vi "Teleop.vi"(10 "Match Info":T1={"Autonomous Elapsed Seconds"=0.0, "TeleOp Elapsed Seconds"=0.0, "Disabled Elapsed Seconds"=0.0, "Visited Autonomous"=FALSE, "Visited TeleOp"=FALSE, "Visited Disabled"=FALSE, "Autonomous Settings"={"Autonomous Style"=enum."Independent", "VI Refnum"=refnum}}, 11 "Call Context":T2) -> ()   [LabVIEW 2016]
doc: "This VI is called for each TeleOp packet received from the DS where the robot is not disabled. It is often used to read from the joysticks and update I/O or to update setpoints for timed control loops. It should complete and return within 20 milliseconds or it may miss DS packets."
uses:
  <vilib>/Rock Robotics/WPI/DriverStation/WPI_DriverStationDerivedRobotMode.ctl
  <vilib>/Rock Robotics/WPI/DriverStation/WPI_DriverStationMatch Info.ctl
  <vilib>/Rock Robotics/WPI/Solenoid/WPI_SolenoidValue.ctl
  <vilib>/Rock Robotics/Network Tables/NT Read Boolean.vi
  <vilib>/Rock Robotics/Network Tables/NT Read Number.vi
  <vilib>/Rock Robotics/WPI/Utilities/WPI_GetSetVariantRefNum.vi
  <vilib>/Rock Robotics/WPI/Solenoid/WPI_SolenoidSetEnum.vi
panel:
  in  "Reset":bool
  out "Teleop Time Elipsed":dbl
  in  "Quand arreter compresseur":dbl
  out "Droit":dbl
  out "Gauche":dbl
  out "Corde start time":dbl
  out "Sample Slider 0":dbl(slide) scale=0.0..5.0
  out "Sample Boolean 1":bool
  out "Sample Boolean 0":bool
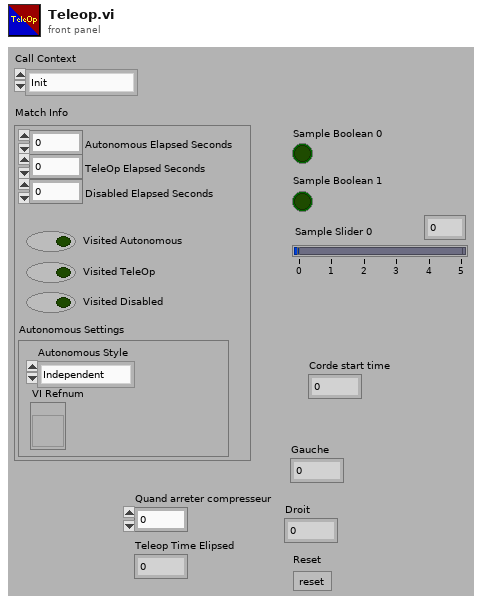
[diagram p1: front panel]
types:
  T1 = typedef "WPI_DriverStationMatch Info.ctl" = cluster{"Autonomous Elapsed Seconds":dbl, "TeleOp Elapsed Seconds":dbl, "Disabled Elapsed Seconds":dbl, "Visited Autonomous":bool, "Visited TeleOp":bool, "Visited Disabled":bool, "Autonomous Settings":cluster{"Autonomous Style":enum16{"Iterative", "Independent"}, "VI Refnum":refnum<vi>}}
  T2 = typedef "WPI_DriverStationDerivedRobotMode.ctl" = enum16{"Init", "Execute", "Stop"}
  T3 = typedef "WPI_SolenoidValue.ctl" = enum16{"Off", "On", "Forward", "Reverse"}
  T4 = typedef "WPI_JoystickDevRef.ctl" = cluster{"Device":T5}
  T5 = typedef "WPI_JoystickDeviceEnum.ctl" = enum16{"USB 0", "USB 1", "USB 2", "USB 3", "USB 4", "USB 5"}
  T6 = typedef "WPI_EncoderDevRef.ctl" = cluster{"DevStatus":errorcluster, "EncoderIndex":T7, "CounterIndex":T8, "DistancePerCount":dbl, "Decoding Type":T9}
  T7 = typedef "FPGA_EncoderIdx.ctl" = enum8{"Enc 0", "Enc 1", "Enc 2", "Enc 3", "Enc 4", "Enc 5", "Enc 6", "Enc 7", "Invalid"}
  T8 = typedef "FPGA_CounterCtrSystemIndex.ctl" = enum8{"Ctr 0", "Ctr 1", "Ctr 2", "Ctr 3", "Ctr 4", "Ctr 5", "Ctr 6", "Ctr 7", "Invalid"}
  T9 = typedef "WPI_EncoderType.ctl" = enum16{"1x", "2x", "4x"}
  T10 = cluster{"Buttons[0]":bool, "Buttons[1]":bool, "Buttons[2]":bool, "Buttons[3]":bool, "Buttons[4]":bool, "Buttons[5]":bool, "Buttons[6]":bool, "Buttons[7]":bool, "Buttons[8]":bool}
  T11 = cluster{"Axes[0]":dbl, "Axes[1]":dbl, "Axes[2]":dbl, "Axes[3]":dbl, "Axes[4]":dbl, "Axes[5]":dbl, "Axes[6]":dbl, "Axes[7]":dbl, "Axes[8]":dbl}
  T12 = typedef "WPI_MotorControlDeviceRef.ctl" = cluster{"DeviceStatus":errorcluster, "Type":T13, "PWM":cluster{"PWM Channel":T14, "DeadBand":T15}, "CAN":cluster{"Device Number":u8, "SetOutput VI Ref":variant, "GetOutput VI Ref":variant, "Enable VI Ref":variant, "Disable VI Ref":variant, "Data":variant}, "Invert":bool}
  T13 = typedef "WPI_MotorControlType.ctl" = enum16{"PWM", "CAN"}
  T14 = typedef "FPGA_DIOPWMChannel.ctl" = enum8{"PWM 0", "PWM 1", "PWM 2", "PWM 3", "PWM 4", "PWM 5", "PWM 6", "PWM 7", "PWM 8", "PWM 9", "PWM MXP 0", "PWM MXP 1", "PWM MXP 2", "PWM MXP 3", "PWM MXP 4", "PWM MXP 5", "PWM MXP 6", "PWM MXP 7", "PWM MXP 8", "PWM MXP 9", "Invalid"}
  T15 = typedef "WPI_PWMDeadband.ctl" = cluster{"Name":string, "maxPositivePwm":i32, "minPositivePwm":i32, "centerPwm":i32, "maxNegativePwm":i32, "minNegativePwm":i32, "angularRange":u16}
  T16 = typedef "WPI_SolenoidDevRef.ctl" = cluster{"DevStatus":errorcluster, "Pneumatics Control Module":u8, "Forward Solenoid Channel":T17, "Reverse Solenoid Channel":T17}
  T17 = typedef "WPI_SolenoidChannel.ctl" = enum8{"Solenoid 0", "Solenoid 1", "Solenoid 2", "Solenoid 3", "Solenoid 4", "Solenoid 5", "Solenoid 6", "Solenoid 7", "Invalid"}
  T18 = typedef "WPI_RobotDriveDevRef.ctl" = cluster{"DevStatus":errorcluster, "Motors[]":T12[], "Square Inputs":bool, "Max Output":dbl}
  T19 = typedef "WPI_CompressorDevRef.ctl" = cluster{"DevStatus":errorcluster, "Pneumatics Control Module":u8}
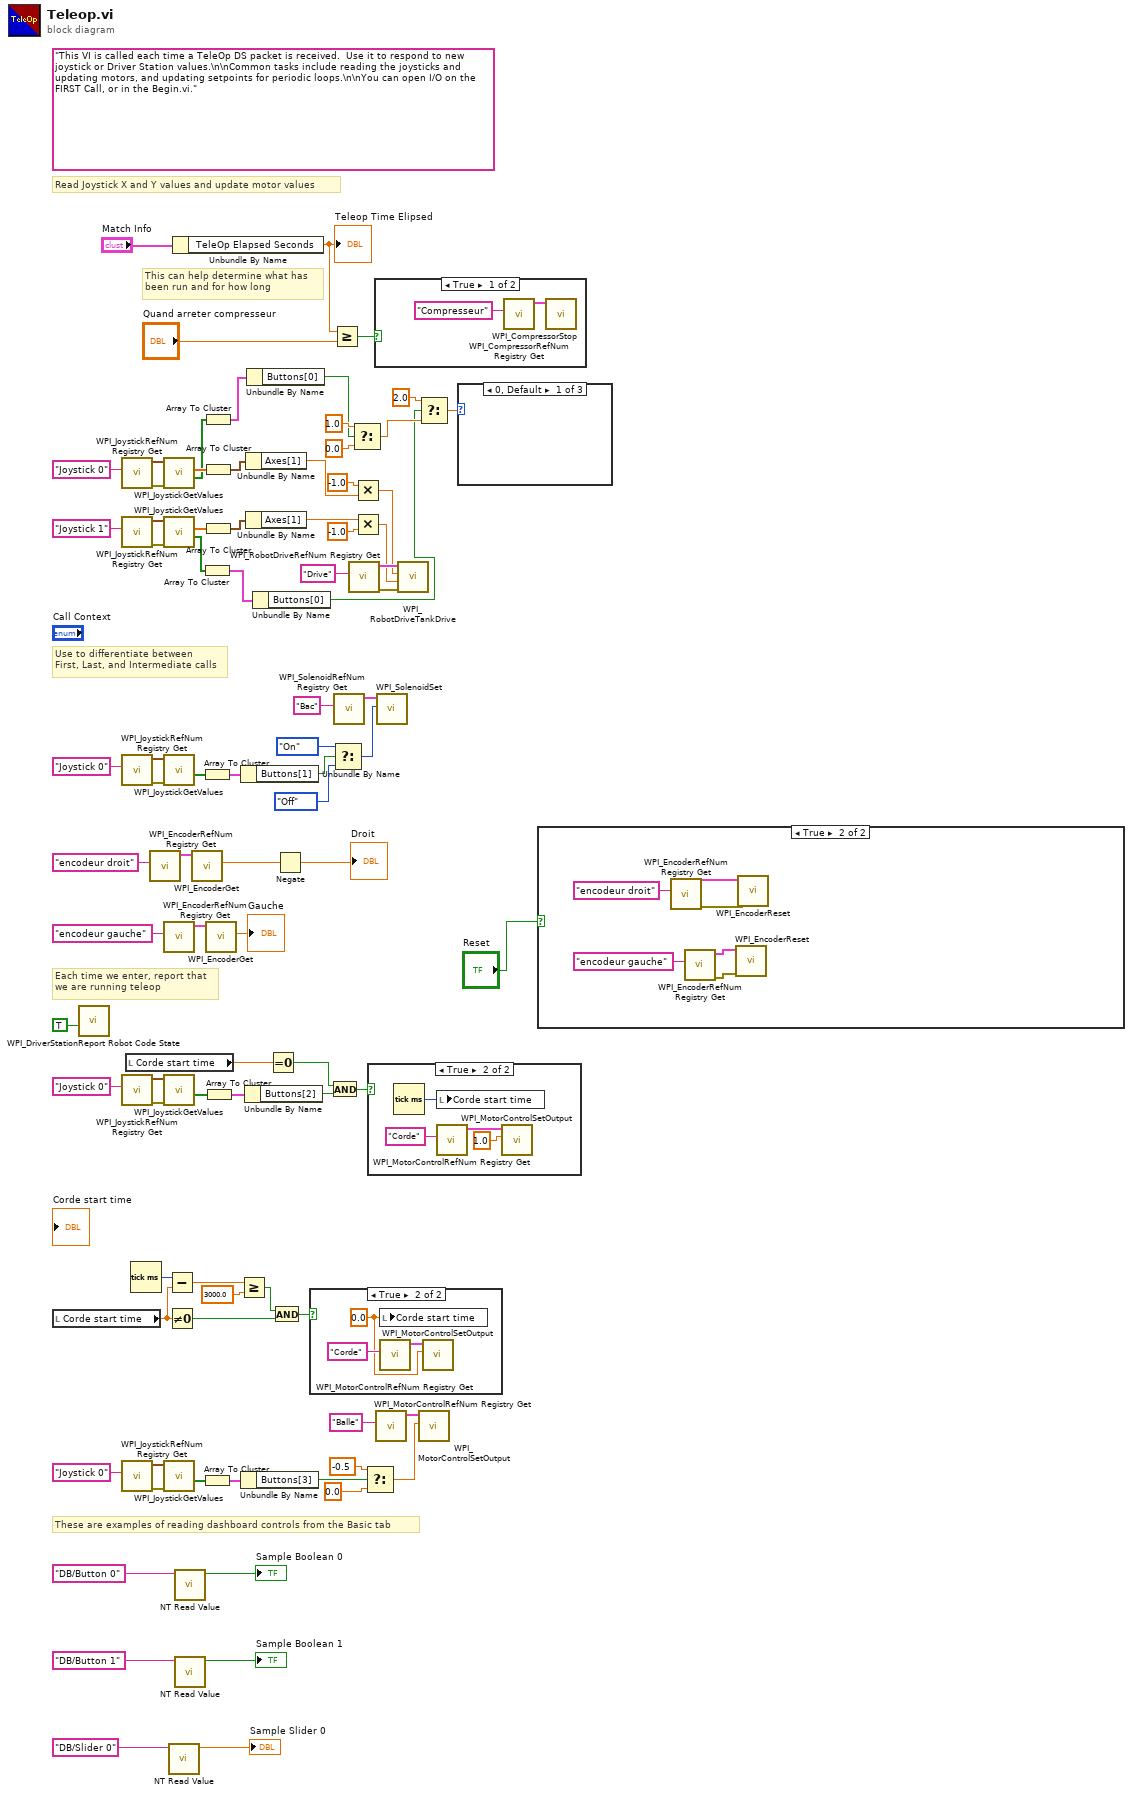
[diagram p0: block diagram]
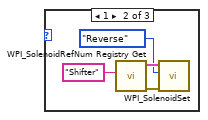
[diagram p6: hidden frame]
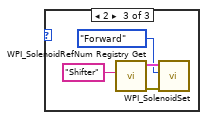
[diagram p7: hidden frame]
diagram:
  (unwired) "This VI is called each time a TeleOp DS packet is received.  Use it to respond to new joystick or Driver Station values.\n\nCommon tasks include reading the joysticks and updating motors, and updating setpoints for periodic loops.\n\nYou can open I/O on the FIRST Call, or in the Begin.vi."
  # "These are examples of reading dashboard controls from the Basic tab"
  # "Each time we enter, report that\nwe are running teleop"
  # "Use to differentiate between\nFirst, Last, and Intermediate calls"
  # "This can help determine what has\nbeen run and for how long"
  # "Read Joystick X and Y values and update motor values"
  n1 = local read "Corde start time"() -> (w28:dbl)
  n2 = call <vilib>:"WPI_DriverStationReport Robot Code State.vi"("TeleOp"=TRUE ("Autonomous")) -> ()  [unwired: 10 in, 1 out]
  n3 = call <vilib>:"WPI_JoystickRefNum Registry Get.vi"("refnum name"="Joystick 0") -> ("error out"=w76:errorcluster, "JoystickDevRef"=w75:T4)  [unwired: 9 in]
  n4 = call <vilib>:"WPI_JoystickRefNum Registry Get.vi"("refnum name"="Joystick 1") -> ("error out"=w14:errorcluster, "JoystickDevRef"=w13:T4)  [unwired: 9 in]
  n5 = call <vilib>:"WPI_JoystickRefNum Registry Get.vi"("refnum name"="Joystick 0") -> ("error out"=w63:errorcluster, "JoystickDevRef"=w64:T4)  [unwired: 1 in, 8 out]
  n6 = call <vilib>:"WPI_JoystickRefNum Registry Get.vi"("refnum name"="Joystick 0") -> ("error out"=w52:errorcluster, "JoystickDevRef"=w53:T4)  [unwired: 1 in, 8 out]
  n7 = call <vilib>:"WPI_JoystickRefNum Registry Get.vi"("refnum name"="Joystick 0") -> ("error out"=w47:errorcluster, "JoystickDevRef"=w48:T4)  [unwired: 1 in, 8 out]
  n8 = local read "Corde start time"() -> (w35:dbl)
  n9 = Tick Count (ms)() -> (millisecond timer value=w34:u32)
  n10 = call <vilib>:"WPI_EncoderRefNum Registry Get.vi"("refnum name"="encodeur droit") -> ("EncoderDevRef"=w26:T6)  [unwired: 9 in, 1 out]
  n11 = call <vilib>:"WPI_JoystickGetValues.vi"("error in (no error)"=w76, "JoystickDevRef"=w75) -> ("Buttons"=w71:bool[], "Axes"=w74:dbl[])  [unwired: 5 in, 3 out]
  n12 = call <vilib>:"WPI_JoystickGetValues.vi"("error in (no error)"=w14, "JoystickDevRef"=w13) -> ("Buttons"=w4:bool[], "Axes"=w12:dbl[])  [unwired: 5 in, 3 out]
  n13 = call <vilib>:"WPI_JoystickGetValues.vi"("error in (no error)"=w63, "JoystickDevRef"=w64) -> ("Buttons"=w62:bool[])  [unwired: 5 in, 4 out]
  n14 = call <vilib>:"WPI_EncoderRefNum Registry Get.vi"("refnum name"="encodeur gauche") -> ("EncoderDevRef"=w27:T6)  [unwired: 9 in, 1 out]
  n15 = call <vilib>:"WPI_JoystickGetValues.vi"("error in (no error)"=w52, "JoystickDevRef"=w53) -> ("Buttons"=w51:bool[])  [unwired: 5 in, 4 out]
  n16 = call <vilib>:"WPI_JoystickGetValues.vi"("error in (no error)"=w47, "JoystickDevRef"=w48) -> ("Buttons"=w46:bool[])  [unwired: 5 in, 4 out]
  n17 = Subtract(x=w34, y=w28) -> (x-y=w33:dbl)
  n18 = Not Equal To 0?(x=w28) -> (x != 0?=w30:bool)
  n19 = call-poly <vilib>:"NT Read Value.vi"("Name"="DB/Slider 0" ("refnum name")) -> ("Numeric"=→"Sample Slider 0":dbl)  [unwired: 9 in, 1 out]
  n20 = Unbundle By Name("Match Info") -> ("TeleOp Elapsed Seconds"=w20:dbl)
  "Teleop Time Elipsed" <- w20
  n21 = call-poly <vilib>:"NT Read Value.vi"("Name"="DB/Button 0" ("refnum name")) -> ("Boolean"=→"Sample Boolean 0":bool)  [unwired: 9 in, 1 out]
  n22 = call-poly <vilib>:"NT Read Value.vi"("Name"="DB/Button 1" ("refnum name")) -> ("Boolean"=→"Sample Boolean 1":bool)  [unwired: 9 in, 1 out]
  n23 = call <vilib>:"WPI_EncoderGet.vi"("EncoderDevRef"=w26) -> ("Distance"=w7:dbl)  [unwired: 5 in, 5 out]
  n24 = Array To Cluster(array=w4) -> (cluster=w3:T10)
  n25 = Array To Cluster(array=w62) -> (cluster=w61:T10)
  n26 = Array To Cluster(array=w46) -> (cluster=w45:T10)
  n27 = Array To Cluster(array=w71) -> (cluster=w5:T10)
  n28 = Array To Cluster(array=w74) -> (cluster=w73:T11)
  n29 = Array To Cluster(array=w12) -> (cluster=w11:T11)
  n30 = Array To Cluster(array=w51) -> (cluster=w50:T10)
  n31 = call <vilib>:"WPI_EncoderGet.vi"("EncoderDevRef"=w27) -> ("Distance"=→"Gauche":dbl)  [unwired: 5 in, 5 out]
  n32 = Greater Or Equal?(x=w33, y=3000.0) -> (x >= y?=w29:bool)
  n33 = Unbundle By Name(w61) -> ("Buttons[1]"=w60:bool)
  n34 = Unbundle By Name(w45) -> ("Buttons[3]"=w44:bool)
  n35 = Unbundle By Name(w50) -> ("Buttons[2]"=w37:bool)
  n36 = Unbundle By Name(w73) -> ("Axes[1]"=w19:dbl)
  n37 = Unbundle By Name(w11) -> ("Axes[1]"=w9:dbl)
  n38 = Unbundle By Name(w5) -> ("Buttons[0]"=w2:bool)
  n39 = Unbundle By Name(w3) -> ("Buttons[0]"=w1:bool)
  n40 = Equal To 0?(x=w35) -> (x = 0?=w36:bool)
  n41 = And(x=w29, y=w30) -> (x .and. y?=w31:bool)
  n42 = Negate(x=w7) -> (-x=→"Droit":dbl)
  n43 = case shown="True" w31 {
    frame False {
    }
    frame True {
      w88 = 0.0 ("Corde start time")
      n44 = local write "Corde start time"(w88) -> ()
      n45 = call <vilib>:"WPI_MotorControlRefNum Registry Get.vi"("refnum name"="Corde") -> ("MotorControlDevRef"=w90:T12)  [unwired: 9 in, 1 out]
      n46 = call <vilib>:"WPI_MotorControlSetOutput.vi"("Output"=w88, "MotorControlDevRef"=w90) -> ()  [unwired: 7 in, 3 out]
    }
  }
  n47 = And(x=w36, y=w37) -> (x .and. y?=w38:bool)
  n48 = Greater Or Equal?(x=w20, y="Quand arreter compresseur") -> (x >= y?=w21:bool)
  n49 = Select(t=WPI_SolenoidValue."On" ("Value"), s=w60, f=WPI_SolenoidValue."Off" ("Value")) -> (s? t:f=w55:T3)
  n50 = call <vilib>:"WPI_SolenoidRefNum Registry Get.vi"("refnum name"="Bac") -> ("SolenoidDevRef"=w56:T16)  [unwired: 9 in, 1 out]
  n51 = call <vilib>:"WPI_RobotDriveRefNum Registry Get.vi"("refnum name"="Drive") -> ("error out"=w79:errorcluster, "RobotDriveDevRef"=w78:T18)  [unwired: 9 in]
  n52 = Select(t=1.0, s=w2, f=0.0) -> (s? t:f=w69:dbl)
  n53 = Multiply(x=-1.0, y=w19) -> (x*y=w16:dbl)
  n54 = Multiply(x=w9, y=-1.0) -> (x*y=w15:dbl)
  n55 = Select(t=-0.5, s=w44, f=0.0) -> (s? t:f=w41:dbl)
  n56 = case shown="True" w38 {
    frame False {
    }
    frame True {
      n57 = Tick Count (ms)() -> (millisecond timer value=w94:u32)
      n58 = local write "Corde start time"(w94) -> ()
      n59 = call <vilib>:"WPI_MotorControlRefNum Registry Get.vi"("refnum name"="Corde") -> ("MotorControlDevRef"=w93:T12)  [unwired: 9 in, 1 out]
      n60 = call <vilib>:"WPI_MotorControlSetOutput.vi"("Output"=1.0, "MotorControlDevRef"=w93) -> ()  [unwired: 7 in, 3 out]
    }
  }
  n61 = case shown="True" w21 {
    frame True {
      n62 = call <vilib>:"WPI_CompressorRefNum Registry Get.vi"("refnum name"="Compresseur") -> ("CompressorDevRef"=w96:T19)  [unwired: 9 in, 1 out]
      n63 = call <vilib>:"WPI_CompressorStop.vi"("CompressorDevRef"=w96) -> ()  [unwired: 9 in, 2 out]
    }
    frame False {
    }
  }
  n64 = call <vilib>:"WPI_MotorControlRefNum Registry Get.vi"("refnum name"="Balle") -> ("MotorControlDevRef"=w39:T12)  [unwired: 9 in, 1 out]
  n65 = call-poly <vilib>:"WPI_SolenoidSet.vi"("Value"=w55, "SolenoidDevRef"=w56) -> ()  [unwired: 8 in, 2 out]
  n66 = call <vilib>:"WPI_RobotDriveTankDrive.vi"("error in (no error)"=w79, "Right axis value"=w15, "Left axis value"=w16, "RobotDriveDevRef"=w78) -> ()  [unwired: 5 in, 3 out]
  n67 = Select(t=2.0, s=w1, f=w69) -> (s? t:f=w66:dbl)
  n68 = call <vilib>:"WPI_MotorControlSetOutput.vi"("Output"=w41, "MotorControlDevRef"=w39) -> ()  [unwired: 7 in, 3 out]
  n69 = case shown="0, Default" w66 {
    frame 0, Default {
    }
    frame 1 {
      n70 = call <vilib>:"WPI_SolenoidRefNum Registry Get.vi"("refnum name"="Shifter") -> ("error out"=w99:errorcluster, "SolenoidDevRef"=w98:T16)  [unwired: 9 in]
      n71 = call-poly <vilib>:"WPI_SolenoidSet.vi"("error in (no error)"=w99, "Value"=WPI_SolenoidValue."Reverse", "SolenoidDevRef"=w98) -> ()  [unwired: 7 in, 2 out]
    }
    frame 2 {
      n72 = call <vilib>:"WPI_SolenoidRefNum Registry Get.vi"("refnum name"="Shifter") -> ("error out"=w103:errorcluster, "SolenoidDevRef"=w102:T16)  [unwired: 9 in]
      n73 = call-poly <vilib>:"WPI_SolenoidSet.vi"("error in (no error)"=w103, "Value"=WPI_SolenoidValue."Forward", "SolenoidDevRef"=w102) -> ()  [unwired: 7 in, 2 out]
    }
  }
  n74 = case shown="True" "Reset" {
    frame False {
    }
    frame True {
      n75 = call <vilib>:"WPI_EncoderRefNum Registry Get.vi"("refnum name"="encodeur droit") -> ("error out"=w107:errorcluster, "EncoderDevRef"=w108:T6)  [unwired: 9 in]
      n76 = call <vilib>:"WPI_EncoderRefNum Registry Get.vi"("refnum name"="encodeur gauche") -> ("error out"=w106:errorcluster, "EncoderDevRef"=w105:T6)  [unwired: 9 in]
      n77 = call <vilib>:"WPI_EncoderReset.vi"("error in (no error)"=w106, "EncoderDevRef"=w105) -> ()  [unwired: 8 in, 2 out]
      n78 = call <vilib>:"WPI_EncoderReset.vi"("error in (no error)"=w107, "EncoderDevRef"=w108) -> ()  [unwired: 8 in, 2 out]
    }
  }
